vi "Lab Panel V5.23.vi"() -> ()   [LabVIEW 2013] (continued)
                            n1466 = local write "RESULT LAB04-2"(TRUE) -> ()
                            n1467 = local write "DISP LAB04-2"(w2761) -> ()
                          }
                        }
                      }
                      frame False {
                      }
                    }
                  }
                }
              }
              frame #8 {
                # "LAB05-1"
                n1468 = Equal?(x=w2764, y=2) -> (x = y?=w2767:bool)
                n1469 = local read "DISP LAB05-1"() -> (w2769:T4)
                n1470 = Unbundle(w2769) -> ("STATUS"=w2770:string)  [unwired: 2 out]
                n1471 = Equal?(x=w2770, y="RUN") -> (x = y?=w2766:bool)
                n1472 = And(x=w2766, y=w2767) -> (x .and. y?=w2765:bool)
                n1473 = case shown="True" w2765 {
                  tunnel: w2769 -> [_ w2773]
                  tunnel: w2763 -> [_ w2776]
                  frame False {
                  }
                  frame True {
                    n1474 = local read "SET LAB05-1"() -> (w2775:T5)
                    n1475 = local read "TDMS LAB05-1"() -> (w2772:refnum<k34>)
                    n1476 = Unbundle(w2773) -> ("CYCLE"=w2777:dbl)  [unwired: 2 out]
                    n1477 = Unbundle(w2775) -> ("T-RISE mins"=w2774:dbl)  [unwired: 4 out]
                    n1478 = Greater Or Equal?(x=w2777, y=w2776) -> (x >= y?=w2778:bool)
                    n1479 = case shown="True" w2778 {
                      tunnel: w2774 -> [w2781 _]
                      tunnel: w2773 -> [w2780 _]
                      tunnel: w2772 -> [w2779 _]
                      frame True {
                        n1480 = stacked-sequence {
                          tunnel: w2781 -> [w2784 _]
                          tunnel: w2780 -> [_ w2789]
                          tunnel: w2779 -> [w2782 _]
                          frame #0 {
                            n1481 = Build Array("T-RISE") -> (w2786:string[])
                            n1482 = Build Array(w2784) -> (w2785:dbl[])
                            n1483 = TDMS Write(0:w2782, 5:"TEST PASS", 7:w2786, 9:w2785) -> (15:w2788:errorcluster)  [unwired: 2 in, 3 out]
                            n1484 = local write "data file error"(w2788) -> ()
                          }
                          frame #1 {
                            n1485 = Bundle(cluster=w2789, "STATUS"="T-RISE PASS") -> (w2791:T4)  [unwired: 2 in]
                            n1486 = local write "RESULT LAB05-1"(TRUE) -> ()
                            n1487 = local write "DISP LAB05-1"(w2791) -> ()
                          }
                        }
                      }
                      frame False {
                      }
                    }
                  }
                }
              }
              frame #9 {
                # "LAB05-2"
                n1488 = Equal?(x=w2794, y=2) -> (x = y?=w2797:bool)
                n1489 = local read "DISP LAB05-2"() -> (w2799:T4)
                n1490 = Unbundle(w2799) -> ("STATUS"=w2800:string)  [unwired: 2 out]
                n1491 = Equal?(x=w2800, y="RUN") -> (x = y?=w2796:bool)
                n1492 = And(x=w2796, y=w2797) -> (x .and. y?=w2795:bool)
                n1493 = case shown="True" w2795 {
                  tunnel: w2799 -> [_ w2803]
                  tunnel: w2793 -> [_ w2806]
                  frame False {
                  }
                  frame True {
                    n1494 = local read "SET LAB05-2"() -> (w2805:T5)
                    n1495 = local read "TDMS LAB05-2"() -> (w2802:refnum<k34>)
                    n1496 = Unbundle(w2803) -> ("CYCLE"=w2807:dbl)  [unwired: 2 out]
                    n1497 = Unbundle(w2805) -> ("T-RISE mins"=w2804:dbl)  [unwired: 4 out]
                    n1498 = Greater Or Equal?(x=w2807, y=w2806) -> (x >= y?=w2808:bool)
                    n1499 = case shown="True" w2808 {
                      tunnel: w2804 -> [w2811 _]
                      tunnel: w2803 -> [w2810 _]
                      tunnel: w2802 -> [w2809 _]
                      frame True {
                        n1500 = stacked-sequence {
                          tunnel: w2811 -> [w2814 _]
                          tunnel: w2810 -> [_ w2819]
                          tunnel: w2809 -> [w2812 _]
                          frame #0 {
                            n1501 = Build Array("T-RISE") -> (w2816:string[])
                            n1502 = Build Array(w2814) -> (w2815:dbl[])
                            n1503 = TDMS Write(0:w2812, 5:"TEST PASS", 7:w2816, 9:w2815) -> (15:w2818:errorcluster)  [unwired: 2 in, 3 out]
                            n1504 = local write "data file error"(w2818) -> ()
                          }
                          frame #1 {
                            n1505 = Bundle(cluster=w2819, "STATUS"="T-RISE PASS") -> (w2821:T4)  [unwired: 2 in]
                            n1506 = local write "RESULT LAB05-2"(TRUE) -> ()
                            n1507 = local write "DISP LAB05-2"(w2821) -> ()
                          }
                        }
                      }
                      frame False {
                      }
                    }
                  }
                }
              }
            }
          }
          frame #6 {
            # "end test & close test files"
            n1508 = local read "MAIL SETTINGS"() -> (w2827:T7)
            n1509 = Unbundle(w2827) -> ("OUT SERVER ADDRESS"=w2826:string, "FROM ACCOUNT"=w2825:string)  [unwired: 5 out]
            n1510 = stacked-sequence {
              tunnel: w2837 -> [_ _ _ _ _ _ _ _ _ _]
              tunnel: w2838 -> [_ _ _ _ _ _ _ _ _ _]
              tunnel: w2836 -> [_ _ _ _ _ _ _ _ _ _]
              tunnel: w2835 -> [_ _ _ _ _ _ _ _ _ _]
              tunnel: w2834 -> [_ _ _ _ _ _ _ _ _ _]
              tunnel: w2833 -> [_ _ _ _ _ _ _ _ _ _]
              tunnel: w2832 -> [_ _ _ _ _ _ _ _ _ _]
              tunnel: w2831 -> [_ _ _ _ _ _ _ _ _ _]
              tunnel: w2830 -> [_ _ _ _ _ _ _ _ _ _]
              tunnel: w2829 -> [_ _ _ _ _ _ _ _ _ _]
              tunnel: w2826 -> [w2842 w2894 w2942 w2989 w3036 w3083 w3130 w3177 w3224 w3271]
              tunnel: w2825 -> [w2841 w2893 w2941 w2988 w3035 w3082 w3129 w3176 w3223 w3270]
              tunnel: "Mail Test File To:" -> [w2840 w2892 w2940 w2987 w3034 w3081 w3128 w3175 w3222 w3269]
              tunnel: "Mail Test Fail" -> [w2839 w2891 w2939 w2986 w3033 w3080 w3127 w3174 w3221 w3268]
              frame #0 {
                # "LAB01-1"
                n1511 = local read "DISP LAB01-1"() -> (w2846:T4)
                n1512 = local read "run lab01-1"() -> (w2843:bool)
                n1513 = local read "TDMS LAB01-1"() -> (w2844:refnum<k34>)
                n1514 = Unbundle(w2846) -> ("CYCLE"=w2847:dbl, "STATUS"=w2845:string)  [unwired: 1 out]
                n1515 = case shown="True" w2843 {
                  tunnel: w2847 -> [_ w2853]
                  tunnel: w2846 -> [_ w2855]
                  tunnel: w2845 -> [_ w2852]
                  tunnel: w2844 -> [_ w2854]
                  tunnel: w2842 -> [_ w2851]
                  tunnel: w2841 -> [_ w2850]
                  tunnel: w2840 -> [_ w2849]
                  tunnel: w2839 -> [_ w2848]
                  frame False {
                  }
                  frame True {
                    n1516 = Not Equal?(x=w2852, y="RUN") -> (x != y?=w2856:bool)
                    n1517 = Greater?(x=w2853, y=2.0) -> (0:w2858:bool)
                    n1518 = And(x=w2858, y=w2856) -> (x .and. y?=w2857:bool)
                    n1519 = case shown="True" w2857 {
                      tunnel: w2855 -> [_ w2868]
                      tunnel: w2854 -> [_ w2867]
                      tunnel: w2853 -> [_ w2866]
                      tunnel: w2852 -> [_ w2865]
                      tunnel: w2851 -> [_ w2864]
                      tunnel: w2850 -> [_ w2863]
                      tunnel: w2849 -> [_ w2862]
                      tunnel: w2848 -> [_ w2861]
                      frame False {
                      }
                      frame True {
                        n1520 = stacked-sequence {
                          tunnel: w2868 -> [w2872 _ _]
                          tunnel: w2867 -> [_ w2874 _]
                          tunnel: w2866 -> [_ _ _]
                          tunnel: w2865 -> [_ _ w2880]
                          tunnel: w2864 -> [_ _ w2879]
                          tunnel: w2863 -> [_ _ w2878]
                          tunnel: w2862 -> [_ _ w2877]
                          tunnel: w2861 -> [_ _ w2876]
                          frame #0 {
                            w2869 = FALSE
                            n1521 = local write "mail control"("END") -> ()
                            n1522 = Bundle(cluster=w2872) -> (w2871:T4)  [unwired: 3 in]
                            n1523 = local write "DISP LAB01-1"(w2871) -> ()
                            n1524 = local write "O/I  LAB01-1"(w2869) -> ()
                            n1525 = local write "run lab01-1"(w2869) -> ()
                            n1526 = local write "RUN LAB01-1"(w2869) -> ()
                          }
                          frame #1 {
                            n1527 = TDMS Close(11:w2874) -> (0:w2873:errorcluster)  [unwired: 1 in, 1 out]
                            n1528 = local write "data file error"(w2873) -> ()
                          }
                          frame #2 {
                            n1529 = stacked-sequence {
                              tunnel: "LAB01-1" -> [w2882 w2884 _]
                              tunnel: w2880 -> [_ w2890 _]
                              tunnel: w2879 -> [_ w2889 _]
                              tunnel: w2878 -> [_ w2888 _]
                              tunnel: w2877 -> [_ w2887 _]
                              tunnel: w2876 -> [_ w2886 _]
                              frame #0 {
                                n1530 = call "sub vi - defrag tdms v1.vi"("panel id"=w2882) -> ("error out"=w2881:errorcluster)  [unwired: 10 in]
                                n1531 = local write "data file error"(w2881) -> ()
                              }
                              frame #1 {
                                n1532 = Bundle("STATUS"=w2890, "OUT SERVER ADDRESS"=w2889, "FROM ACCOUNT"=w2888, "Mail Test File To:"=w2887, "Mail Test Fail"=w2886) -> (w2883:T26)  [unwired: 1 in]
                                n1533 = call "Save data file (pass-fail) v5.vi"("Input Cluster"=w2883, "panel id"=w2884) -> ("network file save error"=w2885:errorcluster)  [unwired: 8 in, 1 out]
                                n1534 = local write "data file error"(w2885) -> ()
                              }
                              frame #2 {
                              }
                            }
                          }
                        }
                      }
                    }
                  }
                }
              }
              frame #1 {
                # "LAB01-2"
                n1535 = local read "run lab01-2"() -> (w2895:bool)
                n1536 = case shown="True" w2895 {
                  tunnel: w2894 -> [_ w2899]
                  tunnel: w2893 -> [_ w2898]
                  tunnel: w2892 -> [_ w2897]
                  tunnel: w2891 -> [_ w2896]
                  frame False {
                  }
                  frame True {
                    n1537 = local read "DISP LAB01-2"() -> (w2907:T4)
                    n1538 = local read "TDMS LAB01-2"() -> (w2906:refnum<k34>)
                    n1539 = Unbundle(w2907) -> ("CYCLE"=w2901:dbl, "STATUS"=w2900:string)  [unwired: 1 out]
                    n1540 = Not Equal?(x=w2900, y="RUN") -> (x != y?=w2903:bool)
                    n1541 = Greater?(x=w2901, y=2.0) -> (0:w2904:bool)
                    n1542 = And(x=w2904, y=w2903) -> (x .and. y?=w2902:bool)
                    n1543 = case shown="True" w2902 {
                      tunnel: w2907 -> [_ w2916]
                      tunnel: w2906 -> [_ w2915]
                      tunnel: w2901 -> [_ w2914]
                      tunnel: w2900 -> [_ w2913]
                      tunnel: w2899 -> [_ w2912]
                      tunnel: w2898 -> [_ w2911]
                      tunnel: w2897 -> [_ w2910]
                      tunnel: w2896 -> [_ w2909]
                      frame False {
                      }
                      frame True {
                        n1544 = stacked-sequence {
                          tunnel: w2916 -> [w2919 _ _]
                          tunnel: w2915 -> [_ w2921 _]
                          tunnel: w2914 -> [_ _ _]
                          tunnel: w2913 -> [_ _ w2927]
                          tunnel: w2912 -> [_ _ w2926]
                          tunnel: w2911 -> [_ _ w2925]
                          tunnel: w2910 -> [_ _ w2924]
                          tunnel: w2909 -> [_ _ w2923]
                          frame #0 {
                            w2917 = FALSE
                            n1545 = local write "mail control"("END") -> ()
                            n1546 = Bundle(cluster=w2919) -> (w2920:T4)  [unwired: 3 in]
                            n1547 = local write "RUN LAB01-2"(w2917) -> ()
                            n1548 = local write "run lab01-2"(w2917) -> ()
                            n1549 = local write "O/I  LAB01-2"(w2917) -> ()
                            n1550 = local write "DISP LAB01-2"(w2920) -> ()
                          }
                          frame #1 {
                            n1551 = TDMS Close(11:w2921) -> (0:w2922:errorcluster)  [unwired: 1 in, 1 out]
                            n1552 = local write "data file error"(w2922) -> ()
                          }
                          frame #2 {
                            n1553 = stacked-sequence {
                              tunnel: "LAB01-2" -> [w2930 w2931]
                              tunnel: w2927 -> [_ w2936]
                              tunnel: w2926 -> [_ w2935]
                              tunnel: w2925 -> [_ w2934]
                              tunnel: w2924 -> [_ w2933]
                              tunnel: w2923 -> [_ w2932]
                              frame #0 {
                                n1554 = call "sub vi - defrag tdms v1.vi"("panel id"=w2930) -> ("error out"=w2929:errorcluster)  [unwired: 10 in]
                                n1555 = local write "data file error"(w2929) -> ()
                              }
                              frame #1 {
                                n1556 = Bundle("STATUS"=w2936, "OUT SERVER ADDRESS"=w2935, "FROM ACCOUNT"=w2934, "Mail Test File To:"=w2933, "Mail Test Fail"=w2932) -> (w2938:T26)  [unwired: 1 in]
                                n1557 = call "Save data file (pass-fail) v5.vi"("Input Cluster"=w2938, "panel id"=w2931) -> ("network file save error"=w2937:errorcluster)  [unwired: 8 in, 1 out]
                                n1558 = local write "data file error"(w2937) -> ()
                              }
                            }
                          }
                        }
                      }
                    }
                  }
                }
              }
              frame #2 {
                # "LAB02-1"
                n1559 = local read "run lab02-1"() -> (w2943:bool)
                n1560 = case shown="True" w2943 {
                  tunnel: w2942 -> [_ w2947]
                  tunnel: w2941 -> [_ w2946]
                  tunnel: w2940 -> [_ w2945]
                  tunnel: w2939 -> [_ w2944]
                  frame False {
                  }
                  frame True {
                    n1561 = local read "DISP LAB02-1"() -> (w2955:T4)
                    n1562 = Unbundle(w2955) -> ("CYCLE"=w2951:dbl, "STATUS"=w2948:string)  [unwired: 1 out]
                    n1563 = local read "TDMS LAB02-1"() -> (w2954:refnum<k34>)
                    n1564 = Not Equal?(x=w2948, y="RUN") -> (x != y?=w2950:bool)
                    n1565 = Greater?(x=w2951, y=2.0) -> (0:w2952:bool)
                    n1566 = And(x=w2952, y=w2950) -> (x .and. y?=w2949:bool)
                    n1567 = case shown="True" w2949 {
                      tunnel: w2955 -> [_ w2963]
                      tunnel: w2954 -> [_ w2962]
                      tunnel: w2948 -> [_ w2961]
                      tunnel: w2947 -> [_ w2960]
                      tunnel: w2946 -> [_ w2959]
                      tunnel: w2945 -> [_ w2958]
                      tunnel: w2944 -> [_ w2957]
                      frame False {
                      }
                      frame True {
                        n1568 = stacked-sequence {
                          tunnel: w2963 -> [w2966 _ _]
                          tunnel: w2962 -> [_ w2968 _]
                          tunnel: w2961 -> [_ _ w2974]
                          tunnel: w2960 -> [_ _ w2973]
                          tunnel: w2959 -> [_ _ w2972]
                          tunnel: w2958 -> [_ _ w2971]
                          tunnel: w2957 -> [_ _ w2970]
                          frame #0 {
                            w2964 = FALSE
                            n1569 = local write "mail control"("END") -> ()
                            n1570 = Bundle(cluster=w2966) -> (w2967:T4)  [unwired: 3 in]
                            n1571 = local write "O/I  LAB02-1"(w2964) -> ()
                            n1572 = local write "RUN LAB02-1"(w2964) -> ()
                            n1573 = local write "run lab02-1"(w2964) -> ()
                            n1574 = local write "DISP LAB02-1"(w2967) -> ()
                          }
                          frame #1 {
                            n1575 = TDMS Close(11:w2968) -> (0:w2969:errorcluster)  [unwired: 1 in, 1 out]
                            n1576 = local write "data file error"(w2969) -> ()
                          }
                          frame #2 {
                            n1577 = stacked-sequence {
                              tunnel: "LAB02-1" -> [w2977 w2984]
                              tunnel: w2974 -> [_ w2982]
                              tunnel: w2973 -> [_ w2981]
                              tunnel: w2972 -> [_ w2980]
                              tunnel: w2971 -> [_ w2979]
                              tunnel: w2970 -> [_ w2978]
                              frame #0 {
                                n1578 = call "sub vi - defrag tdms v1.vi"("panel id"=w2977) -> ("error out"=w2976:errorcluster)  [unwired: 10 in]
                                n1579 = local write "data file error"(w2976) -> ()
                              }
                              frame #1 {
                                n1580 = Bundle("STATUS"=w2982, "OUT SERVER ADDRESS"=w2981, "FROM ACCOUNT"=w2980, "Mail Test File To:"=w2979, "Mail Test Fail"=w2978) -> (w2983:T26)  [unwired: 1 in]
                                n1581 = call "Save data file (pass-fail) v5.vi"("Input Cluster"=w2983, "panel id"=w2984) -> ("network file save error"=w2985:errorcluster)  [unwired: 8 in, 1 out]
                                n1582 = local write "data file error"(w2985) -> ()
                              }
                            }
                          }
                        }
                      }
                    }
                  }
                }
              }
              frame #3 {
                # "LAB02-2"
                n1583 = local read "run lab02-2"() -> (w2990:bool)
                n1584 = case shown="True" w2990 {
                  tunnel: w2989 -> [_ w2994]
                  tunnel: w2988 -> [_ w2993]
                  tunnel: w2987 -> [_ w2992]
                  tunnel: w2986 -> [_ w2991]
                  frame False {
                  }
                  frame True {
                    n1585 = local read "DISP LAB02-2"() -> (w3002:T4)
                    n1586 = local read "TDMS LAB02-2"() -> (w3001:refnum<k34>)
                    n1587 = Unbundle(w3002) -> ("CYCLE"=w2998:dbl, "STATUS"=w2995:string)  [unwired: 1 out]
                    n1588 = Not Equal?(x=w2995, y="RUN") -> (x != y?=w2997:bool)
                    n1589 = Greater?(x=w2998, y=2.0) -> (0:w2999:bool)
                    n1590 = And(x=w2999, y=w2997) -> (x .and. y?=w2996:bool)
                    n1591 = case shown="True" w2996 {
                      tunnel: w3002 -> [_ w3010]
                      tunnel: w3001 -> [_ w3009]
                      tunnel: w2995 -> [_ w3008]
                      tunnel: w2994 -> [_ w3007]
                      tunnel: w2993 -> [_ w3006]
                      tunnel: w2992 -> [_ w3005]
                      tunnel: w2991 -> [_ w3004]
                      frame False {
                      }
                      frame True {
                        n1592 = stacked-sequence {
                          tunnel: w3010 -> [w3013 _ _]
                          tunnel: w3009 -> [_ w3015 _]
                          tunnel: w3008 -> [_ _ w3021]
                          tunnel: w3007 -> [_ _ w3020]
                          tunnel: w3006 -> [_ _ w3019]
                          tunnel: w3005 -> [_ _ w3018]
                          tunnel: w3004 -> [_ _ w3017]
                          frame #0 {
                            w3011 = FALSE
                            n1593 = local write "mail control"("END") -> ()
                            n1594 = Bundle(cluster=w3013) -> (w3014:T4)  [unwired: 3 in]
                            n1595 = local write "O/I  LAB02-2"(w3011) -> ()
                            n1596 = local write "run lab02-2"(w3011) -> ()
                            n1597 = local write "RUN LAB02-2"(w3011) -> ()
                            n1598 = local write "DISP LAB02-2"(w3014) -> ()
                          }
                          frame #1 {
                            n1599 = TDMS Close(11:w3015) -> (0:w3016:errorcluster)  [unwired: 1 in, 1 out]
                            n1600 = local write "data file error"(w3016) -> ()
                          }
                          frame #2 {
                            n1601 = stacked-sequence {
                              tunnel: "LAB02-2" -> [w3024 w3030]
                              tunnel: w3021 -> [_ w3029]
                              tunnel: w3020 -> [_ w3028]
                              tunnel: w3019 -> [_ w3027]
                              tunnel: w3018 -> [_ w3026]
                              tunnel: w3017 -> [_ w3025]
                              frame #0 {
                                n1602 = call "sub vi - defrag tdms v1.vi"("panel id"=w3024) -> ("error out"=w3023:errorcluster)  [unwired: 10 in]
                                n1603 = local write "data file error"(w3023) -> ()
                              }
                              frame #1 {
                                n1604 = Bundle("STATUS"=w3029, "OUT SERVER ADDRESS"=w3028, "FROM ACCOUNT"=w3027, "Mail Test File To:"=w3026, "Mail Test Fail"=w3025) -> (w3032:T26)  [unwired: 1 in]
                                n1605 = call "Save data file (pass-fail) v5.vi"("Input Cluster"=w3032, "panel id"=w3030) -> ("network file save error"=w3031:errorcluster)  [unwired: 8 in, 1 out]
                                n1606 = local write "data file error"(w3031) -> ()
                              }
                            }
                          }
                        }
                      }
                    }
                  }
                }
              }
              frame #4 {
                # "LAB03-1"
                n1607 = local read "run lab03-1"() -> (w3037:bool)
                n1608 = case shown="True" w3037 {
                  tunnel: w3036 -> [_ w3041]
                  tunnel: w3035 -> [_ w3040]
                  tunnel: w3034 -> [_ w3039]
                  tunnel: w3033 -> [_ w3038]
                  frame False {
                  }
                  frame True {
                    n1609 = local read "DISP LAB03-1"() -> (w3049:T4)
                    n1610 = local read "TDMS LAB03-1"() -> (w3048:refnum<k34>)
                    n1611 = Unbundle(w3049) -> ("CYCLE"=w3045:dbl, "STATUS"=w3042:string)  [unwired: 1 out]
                    n1612 = Not Equal?(x=w3042, y="RUN") -> (x != y?=w3044:bool)
                    n1613 = Greater?(x=w3045, y=2.0) -> (0:w3046:bool)
                    n1614 = And(x=w3046, y=w3044) -> (x .and. y?=w3043:bool)
                    n1615 = case shown="True" w3043 {
                      tunnel: w3049 -> [_ w3057]
                      tunnel: w3048 -> [_ w3056]
                      tunnel: w3042 -> [_ w3055]
                      tunnel: w3041 -> [_ w3054]
                      tunnel: w3040 -> [_ w3053]
                      tunnel: w3039 -> [_ w3052]
                      tunnel: w3038 -> [_ w3051]
                      frame False {
                      }
                      frame True {
                        n1616 = stacked-sequence {
                          tunnel: w3057 -> [w3060 _ _]
                          tunnel: w3056 -> [_ w3062 _]
                          tunnel: w3055 -> [_ _ w3068]
                          tunnel: w3054 -> [_ _ w3067]
                          tunnel: w3053 -> [_ _ w3066]
                          tunnel: w3052 -> [_ _ w3065]
                          tunnel: w3051 -> [_ _ w3064]
                          frame #0 {
                            w3058 = FALSE
                            n1617 = local write "mail control"("END") -> ()
                            n1618 = Bundle(cluster=w3060) -> (w3061:T4)  [unwired: 3 in]
                            n1619 = local write "O/I  LAB03-1"(w3058) -> ()
                            n1620 = local write "run lab03-1"(w3058) -> ()
                            n1621 = local write "RUN LAB03-1"(w3058) -> ()
                            n1622 = local write "DISP LAB03-1"(w3061) -> ()
                          }
                          frame #1 {
                            n1623 = TDMS Close(11:w3062) -> (0:w3063:errorcluster)  [unwired: 1 in, 1 out]
                            n1624 = local write "data file error"(w3063) -> ()
                          }
                          frame #2 {
                            n1625 = stacked-sequence {
                              tunnel: "LAB03-1" -> [w3071 w3077]
                              tunnel: w3068 -> [_ w3076]
                              tunnel: w3067 -> [_ w3075]
                              tunnel: w3066 -> [_ w3074]
                              tunnel: w3065 -> [_ w3073]
                              tunnel: w3064 -> [_ w3072]
                              frame #0 {
                                n1626 = call "sub vi - defrag tdms v1.vi"("panel id"=w3071) -> ("error out"=w3070:errorcluster)  [unwired: 10 in]
                                n1627 = local write "data file error"(w3070) -> ()
                              }
                              frame #1 {
                                n1628 = Bundle("STATUS"=w3076, "OUT SERVER ADDRESS"=w3075, "FROM ACCOUNT"=w3074, "Mail Test File To:"=w3073, "Mail Test Fail"=w3072) -> (w3079:T26)  [unwired: 1 in]
                                n1629 = call "Save data file (pass-fail) v5.vi"("Input Cluster"=w3079, "panel id"=w3077) -> ("network file save error"=w3078:errorcluster)  [unwired: 8 in, 1 out]
                                n1630 = local write "data file error"(w3078) -> ()
                              }
                            }
                          }
                        }
                      }
                    }
                  }
                }
              }
              frame #5 {
                # "LAB03-2"
                n1631 = local read "run lab03-2"() -> (w3084:bool)
                n1632 = case shown="True" w3084 {
                  tunnel: w3083 -> [_ w3088]
                  tunnel: w3082 -> [_ w3087]
                  tunnel: w3081 -> [_ w3086]
                  tunnel: w3080 -> [_ w3085]
                  frame False {
                  }
                  frame True {
                    n1633 = local read "DISP LAB03-2"() -> (w3096:T4)
                    n1634 = Unbundle(w3096) -> ("CYCLE"=w3092:dbl, "STATUS"=w3089:string)  [unwired: 1 out]
                    n1635 = local read "TDMS LAB03-2"() -> (w3095:refnum<k34>)
                    n1636 = Not Equal?(x=w3089, y="RUN") -> (x != y?=w3091:bool)
                    n1637 = Greater?(x=w3092, y=2.0) -> (0:w3093:bool)
                    n1638 = And(x=w3093, y=w3091) -> (x .and. y?=w3090:bool)
                    n1639 = case shown="True" w3090 {
                      tunnel: w3096 -> [_ w3104]
                      tunnel: w3095 -> [_ w3103]
                      tunnel: w3089 -> [_ w3102]
                      tunnel: w3088 -> [_ w3101]
                      tunnel: w3087 -> [_ w3100]
                      tunnel: w3086 -> [_ w3099]
                      tunnel: w3085 -> [_ w3098]
                      frame False {
                      }
                      frame True {
                        n1640 = stacked-sequence {
                          tunnel: w3104 -> [w3107 _ _]
                          tunnel: w3103 -> [_ w3109 _]
                          tunnel: w3102 -> [_ _ w3115]
                          tunnel: w3101 -> [_ _ w3114]
                          tunnel: w3100 -> [_ _ w3113]
                          tunnel: w3099 -> [_ _ w3112]
                          tunnel: w3098 -> [_ _ w3111]
                          frame #0 {
                            w3105 = FALSE
                            n1641 = local write "mail control"("END") -> ()
                            n1642 = Bundle(cluster=w3107) -> (w3108:T4)  [unwired: 3 in]
                            n1643 = local write "RUN LAB03-2"(w3105) -> ()
                            n1644 = local write "O/I  LAB03-2"(w3105) -> ()
                            n1645 = local write "DISP LAB03-2"(w3108) -> ()
                            n1646 = local write "run lab03-2"(w3105) -> ()
                          }
                          frame #1 {
                            n1647 = TDMS Close(11:w3109) -> (0:w3110:errorcluster)  [unwired: 1 in, 1 out]
                            n1648 = local write "data file error"(w3110) -> ()
                          }
                          frame #2 {
                            n1649 = stacked-sequence {
                              tunnel: "LAB03-2" -> [w3118 w3119]
                              tunnel: w3115 -> [_ w3124]
                              tunnel: w3114 -> [_ w3123]
                              tunnel: w3113 -> [_ w3122]
                              tunnel: w3112 -> [_ w3121]
                              tunnel: w3111 -> [_ w3120]
                              frame #0 {
                                n1650 = call "sub vi - defrag tdms v1.vi"("panel id"=w3118) -> ("error out"=w3117:errorcluster)  [unwired: 10 in]
                                n1651 = local write "data file error"(w3117) -> ()
                              }
                              frame #1 {
                                n1652 = Bundle("STATUS"=w3124, "OUT SERVER ADDRESS"=w3123, "FROM ACCOUNT"=w3122, "Mail Test File To:"=w3121, "Mail Test Fail"=w3120) -> (w3126:T26)  [unwired: 1 in]
                                n1653 = call "Save data file (pass-fail) v5.vi"("Input Cluster"=w3126, "panel id"=w3119) -> ("network file save error"=w3125:errorcluster)  [unwired: 8 in, 1 out]
                                n1654 = local write "data file error"(w3125) -> ()
                              }
                            }
                          }
                        }
                      }
                    }
                  }
                }
              }
              frame #6 {
                # "LAB04-1"
                n1655 = local read "run lab04-1"() -> (w3131:bool)
                n1656 = case shown="True" w3131 {
                  tunnel: w3130 -> [_ w3135]
                  tunnel: w3129 -> [_ w3134]
                  tunnel: w3128 -> [_ w3133]
                  tunnel: w3127 -> [_ w3132]
                  frame False {
                  }
                  frame True {
                    n1657 = local read "DISP LAB04-1"() -> (w3143:T4)
                    n1658 = Unbundle(w3143) -> ("CYCLE"=w3139:dbl, "STATUS"=w3136:string)  [unwired: 1 out]
                    n1659 = local read "TDMS LAB04-1"() -> (w3142:refnum<k34>)
                    n1660 = Not Equal?(x=w3136, y="RUN") -> (x != y?=w3138:bool)
                    n1661 = Greater?(x=w3139, y=2.0) -> (0:w3140:bool)
                    n1662 = And(x=w3140, y=w3138) -> (x .and. y?=w3137:bool)
                    n1663 = case shown="True" w3137 {
                      tunnel: w3143 -> [_ w3151]
                      tunnel: w3142 -> [_ w3150]
                      tunnel: w3136 -> [_ w3149]
                      tunnel: w3135 -> [_ w3148]
                      tunnel: w3134 -> [_ w3147]
                      tunnel: w3133 -> [_ w3146]
                      tunnel: w3132 -> [_ w3145]
                      frame False {
                      }
                      frame True {
                        n1664 = stacked-sequence {
                          tunnel: w3151 -> [w3154 _ _]
                          tunnel: w3150 -> [_ w3156 _]
                          tunnel: w3149 -> [_ _ w3162]
                          tunnel: w3148 -> [_ _ w3161]
                          tunnel: w3147 -> [_ _ w3160]
                          tunnel: w3146 -> [_ _ w3159]
                          tunnel: w3145 -> [_ _ w3158]
                          frame #0 {
                            w3152 = FALSE
                            n1665 = local write "mail control"("END") -> ()
                            n1666 = Bundle(cluster=w3154) -> (w3155:T4)  [unwired: 3 in]
                            n1667 = local write "RUN LAB04-1"(w3152) -> ()
                            n1668 = local write "O/I  LAB04-1"(w3152) -> ()
                            n1669 = local write "run lab04-1"(w3152) -> ()
                            n1670 = local write "DISP LAB04-1"(w3155) -> ()
                          }
                          frame #1 {
                            n1671 = TDMS Close(11:w3156) -> (0:w3157:errorcluster)  [unwired: 1 in, 1 out]
                            n1672 = local write "data file error"(w3157) -> ()
                          }
                          frame #2 {
                            n1673 = stacked-sequence {
                              tunnel: "LAB04-1" -> [w3165 w3166]
                              tunnel: w3162 -> [_ w3171]
                              tunnel: w3161 -> [_ w3170]
                              tunnel: w3160 -> [_ w3169]
                              tunnel: w3159 -> [_ w3168]
                              tunnel: w3158 -> [_ w3167]
                              frame #0 {
                                n1674 = call "sub vi - defrag tdms v1.vi"("panel id"=w3165) -> ("error out"=w3164:errorcluster)  [unwired: 10 in]
                                n1675 = local write "data file error"(w3164) -> ()
                              }
                              frame #1 {
                                n1676 = Bundle("STATUS"=w3171, "OUT SERVER ADDRESS"=w3170, "FROM ACCOUNT"=w3169, "Mail Test File To:"=w3168, "Mail Test Fail"=w3167) -> (w3173:T26)  [unwired: 1 in]
                                n1677 = call "Save data file (pass-fail) v5.vi"("Input Cluster"=w3173, "panel id"=w3166) -> ("network file save error"=w3172:errorcluster)  [unwired: 8 in, 1 out]
                                n1678 = local write "data file error"(w3172) -> ()
                              }
                            }
                          }
                        }
                      }
                    }
                  }
                }
              }
              frame #7 {
                # "LAB04-2"
                n1679 = local read "run lab04-2"() -> (w3178:bool)
                n1680 = case shown="True" w3178 {
                  tunnel: w3177 -> [_ w3182]
                  tunnel: w3176 -> [_ w3181]
                  tunnel: w3175 -> [_ w3180]
                  tunnel: w3174 -> [_ w3179]
                  frame False {
                  }
                  frame True {
                    n1681 = local read "DISP LAB04-2"() -> (w3190:T4)
                    n1682 = Unbundle(w3190) -> ("CYCLE"=w3186:dbl, "STATUS"=w3183:string)  [unwired: 1 out]
                    n1683 = Not Equal?(x=w3183, y="RUN") -> (x != y?=w3185:bool)
                    n1684 = local read "TDMS LAB04-2"() -> (w3189:refnum<k34>)
                    n1685 = Greater?(x=w3186, y=2.0) -> (0:w3187:bool)
                    n1686 = And(x=w3187, y=w3185) -> (x .and. y?=w3184:bool)
                    n1687 = case shown="True" w3184 {
                      tunnel: w3190 -> [_ w3198]
                      tunnel: w3189 -> [_ w3197]
                      tunnel: w3183 -> [_ w3196]
                      tunnel: w3182 -> [_ w3195]
                      tunnel: w3181 -> [_ w3194]
                      tunnel: w3180 -> [_ w3193]
                      tunnel: w3179 -> [_ w3192]
                      frame False {
                      }
                      frame True {
                        n1688 = stacked-sequence {
                          tunnel: w3198 -> [w3201 _ _]
                          tunnel: w3197 -> [_ w3203 _]
                          tunnel: w3196 -> [_ _ w3209]
                          tunnel: w3195 -> [_ _ w3208]
                          tunnel: w3194 -> [_ _ w3207]
                          tunnel: w3193 -> [_ _ w3206]
                          tunnel: w3192 -> [_ _ w3205]
                          frame #0 {
                            w3199 = FALSE
                            n1689 = local write "mail control"("END") -> ()
                            n1690 = Bundle(cluster=w3201) -> (w3202:T4)  [unwired: 3 in]
                            n1691 = local write "O/I  LAB04-2"(w3199) -> ()
                            n1692 = local write "RUN LAB04-2"(w3199) -> ()
                            n1693 = local write "run lab04-2"(w3199) -> ()
                            n1694 = local write "DISP LAB04-2"(w3202) -> ()
                          }
                          frame #1 {
                            n1695 = TDMS Close(11:w3203) -> (0:w3204:errorcluster)  [unwired: 1 in, 1 out]
                            n1696 = local write "data file error"(w3204) -> ()
                          }
                          frame #2 {
                            n1697 = stacked-sequence {
                              tunnel: "LAB04-2" -> [w3212 w3213]
                              tunnel: w3209 -> [_ w3218]
                              tunnel: w3208 -> [_ w3217]
                              tunnel: w3207 -> [_ w3216]
                              tunnel: w3206 -> [_ w3215]
                              tunnel: w3205 -> [_ w3214]
                              frame #0 {
                                n1698 = call "sub vi - defrag tdms v1.vi"("panel id"=w3212) -> ("error out"=w3211:errorcluster)  [unwired: 10 in]
                                n1699 = local write "data file error"(w3211) -> ()
                              }
                              frame #1 {
                                n1700 = Bundle("STATUS"=w3218, "OUT SERVER ADDRESS"=w3217, "FROM ACCOUNT"=w3216, "Mail Test File To:"=w3215, "Mail Test Fail"=w3214) -> (w3220:T26)  [unwired: 1 in]
                                n1701 = call "Save data file (pass-fail) v5.vi"("Input Cluster"=w3220, "panel id"=w3213) -> ("network file save error"=w3219:errorcluster)  [unwired: 8 in, 1 out]
                                n1702 = local write "data file error"(w3219) -> ()
                              }
                            }
                          }
                        }
                      }
                    }
                  }
                }
              }
              frame #8 {
                # "LAB05-1"
                n1703 = local read "run lab05-1"() -> (w3225:bool)
                n1704 = case shown="True" w3225 {
                  tunnel: w3224 -> [_ w3229]
                  tunnel: w3223 -> [_ w3228]
                  tunnel: w3222 -> [_ w3227]
                  tunnel: w3221 -> [_ w3226]
                  frame False {
                  }
                  frame True {
                    n1705 = local read "DISP LAB05-1"() -> (w3237:T4)
                    n1706 = Unbundle(w3237) -> ("CYCLE"=w3233:dbl, "STATUS"=w3230:string)  [unwired: 1 out]
                    n1707 = Not Equal?(x=w3230, y="RUN") -> (x != y?=w3232:bool)
                    n1708 = local read "TDMS LAB05-1"() -> (w3236:refnum<k34>)
                    n1709 = Greater?(x=w3233, y=2.0) -> (0:w3234:bool)
                    n1710 = And(x=w3234, y=w3232) -> (x .and. y?=w3231:bool)
                    n1711 = case shown="True" w3231 {
                      tunnel: w3237 -> [_ w3245]
                      tunnel: w3236 -> [_ w3244]
                      tunnel: w3230 -> [_ w3243]
                      tunnel: w3229 -> [_ w3242]
                      tunnel: w3228 -> [_ w3241]
                      tunnel: w3227 -> [_ w3240]
                      tunnel: w3226 -> [_ w3239]
                      frame False {
                      }
                      frame True {
                        n1712 = stacked-sequence {
                          tunnel: w3245 -> [w3248 _ _]
                          tunnel: w3244 -> [_ w3250 _]
                          tunnel: w3243 -> [_ _ w3256]
                          tunnel: w3242 -> [_ _ w3255]
                          tunnel: w3241 -> [_ _ w3254]
                          tunnel: w3240 -> [_ _ w3253]
                          tunnel: w3239 -> [_ _ w3252]
                          frame #0 {
                            w3246 = FALSE
                            n1713 = local write "mail control"("END") -> ()
                            n1714 = Bundle(cluster=w3248) -> (w3249:T4)  [unwired: 3 in]
                            n1715 = local write "O/I  LAB05-1"(w3246) -> ()
                            n1716 = local write "RUN LAB05-1"(w3246) -> ()
                            n1717 = local write "run lab05-1"(w3246) -> ()
                            n1718 = local write "DISP LAB05-1"(w3249) -> ()
                          }
                          frame #1 {
                            n1719 = TDMS Close(11:w3250) -> (0:w3251:errorcluster)  [unwired: 1 in, 1 out]
                            n1720 = local write "data file error"(w3251) -> ()
                          }
                          frame #2 {
                            n1721 = stacked-sequence {
                              tunnel: "LAB05-1" -> [w3259 w3265]
                              tunnel: w3256 -> [_ w3264]
                              tunnel: w3255 -> [_ w3263]
                              tunnel: w3254 -> [_ w3262]
                              tunnel: w3253 -> [_ w3261]
                              tunnel: w3252 -> [_ w3260]
                              frame #0 {
                                n1722 = call "sub vi - defrag tdms v1.vi"("panel id"=w3259) -> ("error out"=w3258:errorcluster)  [unwired: 10 in]
                                n1723 = local write "data file error"(w3258) -> ()
                              }
                              frame #1 {
                                n1724 = Bundle("STATUS"=w3264, "OUT SERVER ADDRESS"=w3263, "FROM ACCOUNT"=w3262, "Mail Test File To:"=w3261, "Mail Test Fail"=w3260) -> (w3267:T26)  [unwired: 1 in]
                                n1725 = call "Save data file (pass-fail) v5.vi"("Input Cluster"=w3267, "panel id"=w3265) -> ("network file save error"=w3266:errorcluster)  [unwired: 8 in, 1 out]
                                n1726 = local write "data file error"(w3266) -> ()
                              }
                            }
                          }
                        }
                      }
                    }
                  }
                }
              }
              frame #9 {
                # "LAB05-2"
                n1727 = local read "run lab05-2"() -> (w3272:bool)
                n1728 = case shown="True" w3272 {
                  tunnel: w3271 -> [_ w3276]
                  tunnel: w3270 -> [_ w3275]
                  tunnel: w3269 -> [_ w3274]
                  tunnel: w3268 -> [_ w3273]
                  frame False {
                  }
                  frame True {
                    n1729 = local read "DISP LAB05-2"() -> (w3284:T4)
                    n1730 = Unbundle(w3284) -> ("CYCLE"=w3280:dbl, "STATUS"=w3277:string)  [unwired: 1 out]
                    n1731 = Not Equal?(x=w3277, y="RUN") -> (x != y?=w3279:bool)
                    n1732 = local read "TDMS LAB05-2"() -> (w3283:refnum<k34>)
                    n1733 = Greater?(x=w3280, y=2.0) -> (0:w3281:bool)
                    n1734 = And(x=w3281, y=w3279) -> (x .and. y?=w3278:bool)
                    n1735 = case shown="True" w3278 {
                      tunnel: w3284 -> [_ w3292]
                      tunnel: w3283 -> [_ w3291]
                      tunnel: w3277 -> [_ w3290]
                      tunnel: w3276 -> [_ w3289]
                      tunnel: w3275 -> [_ w3288]
                      tunnel: w3274 -> [_ w3287]
                      tunnel: w3273 -> [_ w3286]
                      frame False {
                      }
                      frame True {
                        n1736 = stacked-sequence {
                          tunnel: w3292 -> [w3295 _ _]
                          tunnel: w3291 -> [_ w3297 _]
                          tunnel: w3290 -> [_ _ w3303]
                          tunnel: w3289 -> [_ _ w3302]
                          tunnel: w3288 -> [_ _ w3301]
                          tunnel: w3287 -> [_ _ w3300]
                          tunnel: w3286 -> [_ _ w3299]
                          frame #0 {
                            w3293 = FALSE
                            n1737 = local write "mail control"("END") -> ()
                            n1738 = Bundle(cluster=w3295) -> (w3296:T4)  [unwired: 3 in]
                            n1739 = local write "RUN LAB05-2"(w3293) -> ()
                            n1740 = local write "O/I  LAB05-2"(w3293) -> ()
                            n1741 = local write "run lab05-2"(w3293) -> ()
                            n1742 = local write "DISP LAB05-2"(w3296) -> ()
                          }
                          frame #1 {
                            n1743 = TDMS Close(11:w3297) -> (0:w3298:errorcluster)  [unwired: 1 in, 1 out]
                            n1744 = local write "data file error"(w3298) -> ()
                          }
                          frame #2 {
                            n1745 = stacked-sequence {
                              tunnel: "LAB05-2" -> [w3306 w3312]
                              tunnel: w3303 -> [_ w3311]
                              tunnel: w3302 -> [_ w3310]
                              tunnel: w3301 -> [_ w3309]
                              tunnel: w3300 -> [_ w3308]
                              tunnel: w3299 -> [_ w3307]
                              frame #0 {
                                n1746 = call "sub vi - defrag tdms v1.vi"("panel id"=w3306) -> ("error out"=w3305:errorcluster)  [unwired: 10 in]
                                n1747 = local write "data file error"(w3305) -> ()
                              }
                              frame #1 {
                                n1748 = Bundle("STATUS"=w3311, "OUT SERVER ADDRESS"=w3310, "FROM ACCOUNT"=w3309, "Mail Test File To:"=w3308, "Mail Test Fail"=w3307) -> (w3314:T26)  [unwired: 1 in]
                                n1749 = call "Save data file (pass-fail) v5.vi"("Input Cluster"=w3314, "panel id"=w3312) -> ("network file save error"=w3313:errorcluster)  [unwired: 8 in, 1 out]
                                n1750 = local write "data file error"(w3313) -> ()
                              }
                            }
                          }
                        }
                      }
                    }
                  }
                }
              }
            }
            n1751 = local read "Network Directory"() -> (w2828:path)
            n1752 = global write "Global 1.vi" "Network Drive"(w2828) -> ()
          }
          frame #7 {
            # "disable functions"
            n1753 = stacked-sequence {
              tunnel: w3324 -> [w3338 _ w3395]
              tunnel: w3323 -> [w3333 _ w3394]
              tunnel: w3322 -> [w3332 _ w3393]
              tunnel: w3321 -> [w3330 _ w3392]
              tunnel: w3320 -> [w3331 _ w3391]
              tunnel: w3319 -> [_ w3355 w3390]
              tunnel: w3318 -> [_ w3356 w3389]
              tunnel: w3317 -> [_ w3357 w3388]
              tunnel: w3316 -> [_ w3358 w3387]
              tunnel: w3315 -> [_ w3359 w3386]
              frame #0 {
                n1754 = Select(t=2, s=w3330, f=0) -> (s? t:f=w3326:i32)
                n1755 = Select(t=2, s=w3332, f=0) -> (s? t:f=w3327:i32)
                n1756 = Select(t=2, s=w3331, f=0) -> (s? t:f=w3325:i32)
                n1757 = Select(t=2, s=w3338, f=0) -> (s? t:f=w3329:i32)
                n1758 = Select(t=2, s=w3333, f=0) -> (s? t:f=w3328:i32)
                n1759 = property on="SELECT LAB02-2" class="RadioBtnsControl (strict)"("DisabledEnum"=w3326) -> ()  [unwired: 2 in, 2 out]
                n1760 = property on="SELECT LAB02-1" class="RadioBtnsControl (strict)"("DisabledEnum"=w3327) -> ()  [unwired: 2 in, 2 out]
                n1761 = property on="SELECT LAB03-1" class="RadioBtnsControl (strict)"("DisabledEnum"=w3325) -> ()  [unwired: 2 in, 2 out]
